vi "Joystick-triggers.vi"(11 "JoystickDevRef":T1) -> (0 "Right out":dbl, 1 "Left out":dbl, 2 "x+y":dbl, 3 "JoystickDevRef out":T1, 4 "Buttons":bool[](array[boolean]))   [LabVIEW 2015]
uses:
  <vilib>/Rock Robotics/WPI/Joystick/WPI_JoystickDevRef.ctl
  <vilib>/Rock Robotics/WPI/Joystick/WPI_JoystickDeviceEnum.ctl
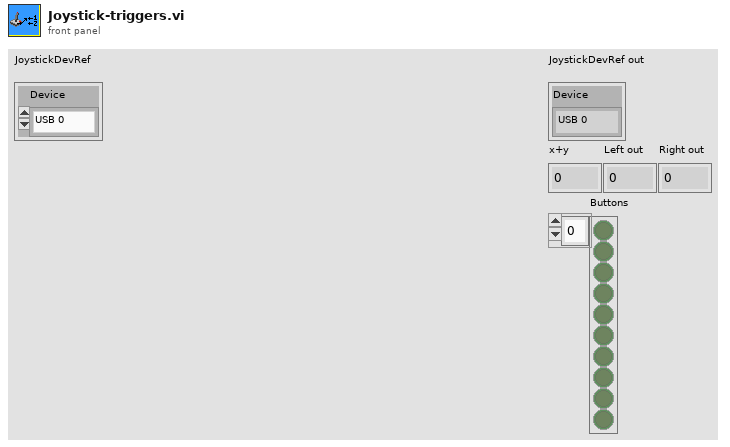
[diagram p1: front panel]
types:
  T1 = typedef "WPI_JoystickDevRef.ctl" = cluster{"Device":T2}
  T2 = typedef "WPI_JoystickDeviceEnum.ctl" = enum16{"USB 0", "USB 1", "USB 2", "USB 3", "USB 4", "USB 5"}
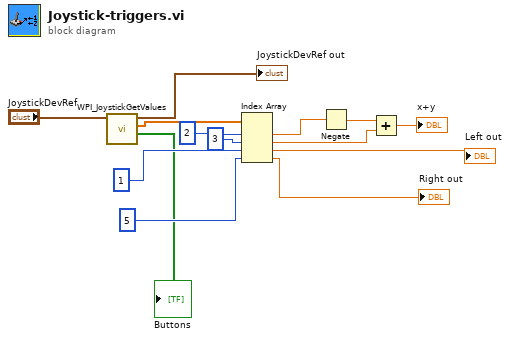
[diagram p0: block diagram]
diagram:
  n1 = call <vilib>:"WPI_JoystickGetValues.vi"("JoystickDevRef"="JoystickDevRef") -> ("Buttons"=→"Buttons":bool[], "Axes"=w12:dbl[], "JoystickDevRef"=→"JoystickDevRef out":T1)  [unwired: 6 in, 2 out]
  n2 = Index Array(array=w12, index #1=2 ("index"), index #2=3 ("index"), index #3=1, index #4=5) -> (element #1=w8:dbl, element #2=w6:dbl, element #3=→"Left out":dbl, element #4=→"Right out":dbl)
  n3 = Negate(x=w8) -> (-x=w9:dbl)
  n4 = Add(x=w9, y=w6) -> (x+y=→"x+y":dbl)
